vi "interp.vi"(1 "first subarray":dbl[](array[numeric]), 2 "nFRAMES":dbl=100.0) -> (0 "emgInterp":dbl[](array[numeric]))   [LabVIEW 2020]
uses:
  <vilib>/Analysis/NI_AALPro.lvlib
panel:
  out "time out sustinhaCrazy":dbl[](array[numeric])
  in  "Type of Interpolation":T1(ring)
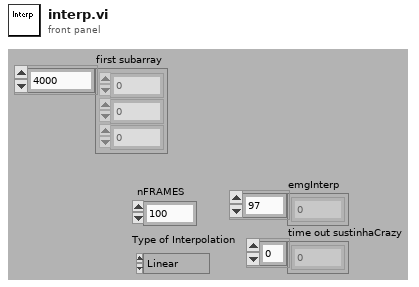
[diagram p1: front panel]
types:
  T1 = enum16{"Linear", "Polynomial", "Spline", "Rational"}
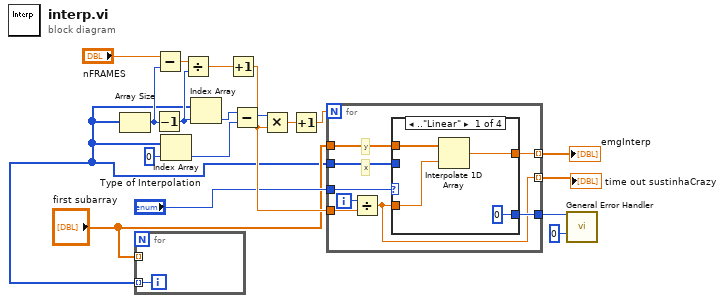
[diagram p0: block diagram]
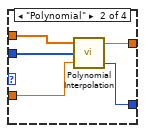
[diagram p2: hidden frame]
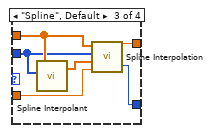
[diagram p3: hidden frame]
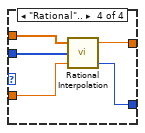
[diagram p4: hidden frame]
diagram:
  n1 = for {
    tunnel: "first subarray" -> [_] mode=indexing
    tunnel: [w20] -> w1 mode=indexing
    i -> [w20]
  }
  n2 = Array Size(array=w1) -> (size(s)=w9:i32)
  n3 = Decrement(x=w9) -> (x-1=w7:i32)
  n4 = Subtract(x="nFRAMES", y=w9) -> (x-y=w6:dbl)
  n5 = Index Array(array=w1, index=0) -> (element=w13:i32)
  n6 = Divide(x=w6, y=w7) -> (x/y=w5:dbl)
  n7 = Index Array(array=w1, index=w7) -> (element=w12:i32)
  n8 = Increment(x=w5) -> (x+1=w11:dbl)
  n9 = Subtract(x=w12, y=w13) -> (x-y=w15:i32)
  n10 = Multiply(x=w15, y=w11) -> (x*y=w16:dbl)
  n11 = Increment(x=w16) -> (x+1=w14:dbl)
  n12 = for {
    N: w14 -> [_]
    tunnel: "first subarray" -> [w28]
    tunnel: w1 -> [w27]
    tunnel: [w26] -> w19
    tunnel: "Type of Interpolation" -> [w21]
    tunnel: w11 -> [w24]
    tunnel: [w23] -> w4 mode=indexing
    tunnel: [w22] -> w3 mode=indexing
    i -> [w25]
    # "x"
    # "y"
    n13 = Divide(x=w25, y=w24) -> (x/y=w22:dbl)
    n14 = case shown="..\"Linear\"" w21 {
      tunnel: w22 -> [w31 w37 w40 w44]
      tunnel: [w30 w36 w38 w46] -> w23
      tunnel: [0 w35 w39 w45] -> w26
      tunnel: w27 -> [_ w34 w41 w47]
      tunnel: w28 -> [w32 w33 w43 w48]
      frame .."Linear" {
        n15 = Interpolate 1D Array(1:w31, 2:w32) -> (0:w30:dbl)
      }
      frame "Polynomial" {
        n16 = call <vilib>:"Polynomial Interpolation.vi"("x value"=w37, "X"=w34, "Y"=w33) -> ("error"=w35:i32, "interpolation value"=w36:dbl)  [unwired: 1 out]
      }
      frame "Spline", Default {
        n17 = call <vilib>:"Spline Interpolant.vi"("X"=w41, "Y"=w43) -> ("Interpolant"=w42:dbl[])  [unwired: 2 in, 1 out]
        n18 = call <vilib>:"Spline Interpolation.vi"("x value"=w40, "Interpolant"=w42, "X"=w41, "Y"=w43) -> ("error"=w39:i32, "interpolation value"=w38:dbl)
      }
      frame "Rational".. {
        n19 = call <vilib>:"Rational Interpolation.vi"("x value"=w44, "X"=w47, "Y"=w48) -> ("error"=w45:i32, "interpolation value"=w46:dbl)  [unwired: 1 out]
      }
    }
  }
  "emgInterp" <- w4
  "time out sustinhaCrazy" <- w3
  n20 = call <vilib>:"General Error Handler.vi"("[error code] (0)"=w19, "type of dialog (OK msg:1)"=0) -> ()  [unwired: 9 in, 5 out]
